vi "Get data sel exp.vi"(8 "error in (no error)":errorcluster, 11 "Control-Client in":refnum<class "Control-Client.lvclass">) -> (0 "error out":errorcluster, 2 "Data":sgl[][](array[numeric]), 3 "Control-Client out":refnum<class "Control-Client.lvclass">)   [LabVIEW 2019, in "Control-Client.lvclass"]
uses:
  Control-Client.lvclass
  Experiments/Experiment.lvclass
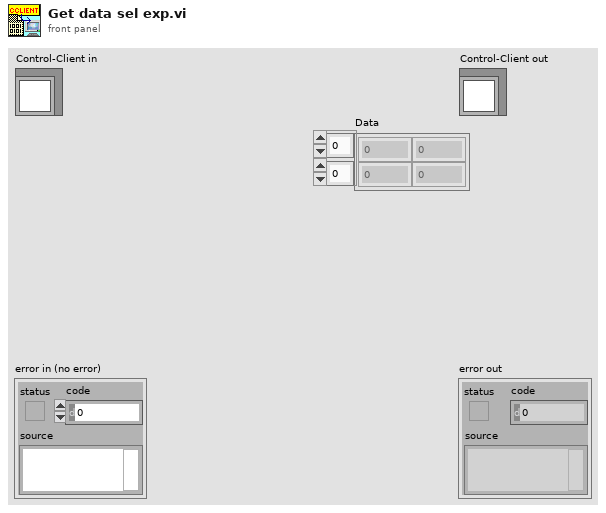
[diagram p1: front panel]
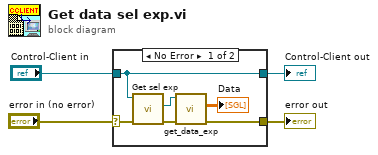
[diagram p0: block diagram]
diagram:
  n1 = case shown="No Error" "error in (no error)" {
    selector: "error in (no error)" -> [w7 w12]
    tunnel: [w5 w12] -> w3
    tunnel: [w8 w11] -> w1
    tunnel: "Control-Client in" -> [w8 w11]
    frame No Error {
      n2 = call "Get sel exp.vi"("error in (no error)"=w7, "Control-Client in"=w8) -> ("error out"=w10:errorcluster, "Sel experiment"=w9:refnum<class "Experiment.lvclass">)  [unwired: 7 in, 1 out]
      n3 = call "get_data_exp.vi"("error in (no error)"=w10, "Experiment.lvclass in"=w9) -> ("error out"=w5:errorcluster, "Data"=→"Data":sgl[][])  [unwired: 7 in, 1 out]
    }
    frame Error {
    }
  }
  "error out" <- w3
  "Control-Client out" <- w1
